vi "Scale signal and truncate below zero values.vi"(9 "Offset":dbl, 10 "Slope":dbl, 11 "Dynamic Data":dynamicdata(waveform)) -> (2 "Un-truncated signal":dynamicdata(waveform), 3 "Truncated signal":dynamicdata(waveform))   [LabVIEW 2016]
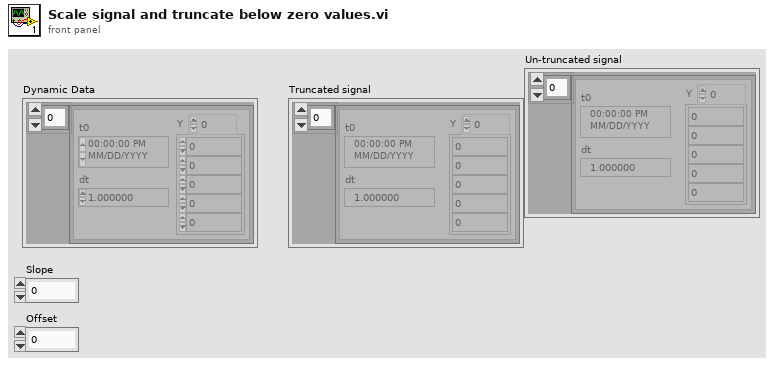
[diagram p1: front panel]
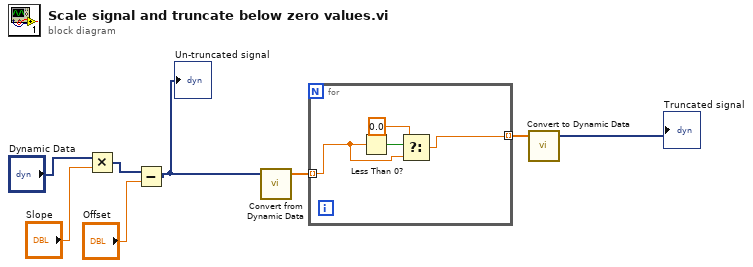
[diagram p0: block diagram]
diagram:
  n1 = Multiply(x="Dynamic Data", y="Slope") -> (x*y=w4:dynamicdata)
  n2 = Subtract(x=w4, y="Offset") -> (x-y=w1:dynamicdata)
  "Un-truncated signal" <- w1
  n3 = call "Convert from Dynamic Data"("Dynamic Data Type"=w1) -> ("Array"=w6:dbl[])  [unwired: 3 in]
  n4 = for {
    tunnel: w6 -> [w9] mode=indexing
    tunnel: [w10] -> w7 mode=indexing
    n5 = Less Than 0?(x=w9) -> (x < 0?=w12:bool)
    n6 = Select(t=0.0, s=w12, f=w9) -> (s? t:f=w10:dbl)
  }
  n7 = call "Convert to Dynamic Data"("Array"=w7) -> ("Dynamic Data Type"=→"Truncated signal":dynamicdata)  [unwired: 3 in]
